vi "质控参数设置.vi"(9 "自动测试量程配置":T1, 10 "质控参数设置":T3) -> (2 "自动测试量程配置输出":T1, 3 "输出簇":T2)   [LabVIEW 2016, in "斯坦道氨氮.lvlib"]
uses:
  <vilib>/Utility/miscctls.llb/LVPointTypeDef.ctl
panel:
  in  "取消":bool
  in  "确定":bool
  in  "总磷标准液标准浓度":dbl
  in  "总磷跨度标准液浓度":dbl
  in  "总磷零点标准液浓度":dbl
  in  "总磷跨度值":dbl
  # "质控量程设置"
  # "监测参数"
  # "氨氮"
  # "跨度值"
  # "mg/L"
  # "零点核查标准液浓度"
  # "mg/L"
  # "跨度核查标准液浓度"
  # "mg/L"
  # "标样核查标准液浓度"
  # "mg/L"
  # "质控参数设置"
  # "监测参数"
  # "氨氮"
  # "跨度值"
  # "零点核查标准液浓度"
  # "跨度核查标准液浓度"
  # "标样核查标准液浓度"
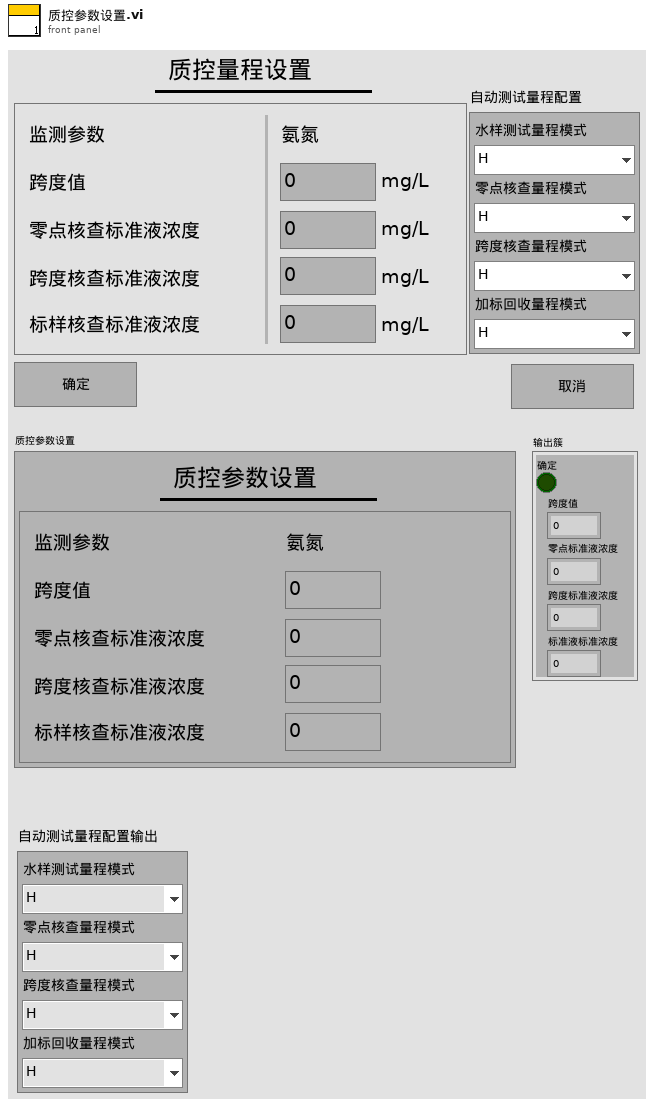
[diagram p1: front panel]
types:
  T1 = cluster{"水样测试量程模式":enum16{"H", "L", "AUTO"}, "空白核查量程模式":enum16{"H", "L", "AUTO"}, "跨度核查量程模式":enum16{"H", "L", "AUTO"}, "加标回收量程模式":enum16{"H", "L", "AUTO"}}
  T2 = cluster{"确定":bool, "跨度值":dbl, "零点标准液浓度":dbl, "跨度标准液浓度":dbl, "标准液标准浓度":dbl}
  T3 = cluster{"总磷跨度值":dbl, "总磷零点标准液浓度":dbl, "总磷跨度标准液浓度":dbl, "总磷标准液标准浓度":dbl}
  T4 = typedef "LVPointTypeDef.ctl" = cluster{"Horizontal":i16, "Vertical":i16}
  T5 = cluster{"确定":bool, "总磷跨度值":dbl, "总磷零点标准液浓度":dbl, "总磷跨度标准液浓度":dbl, "总磷标准液标准浓度":dbl}
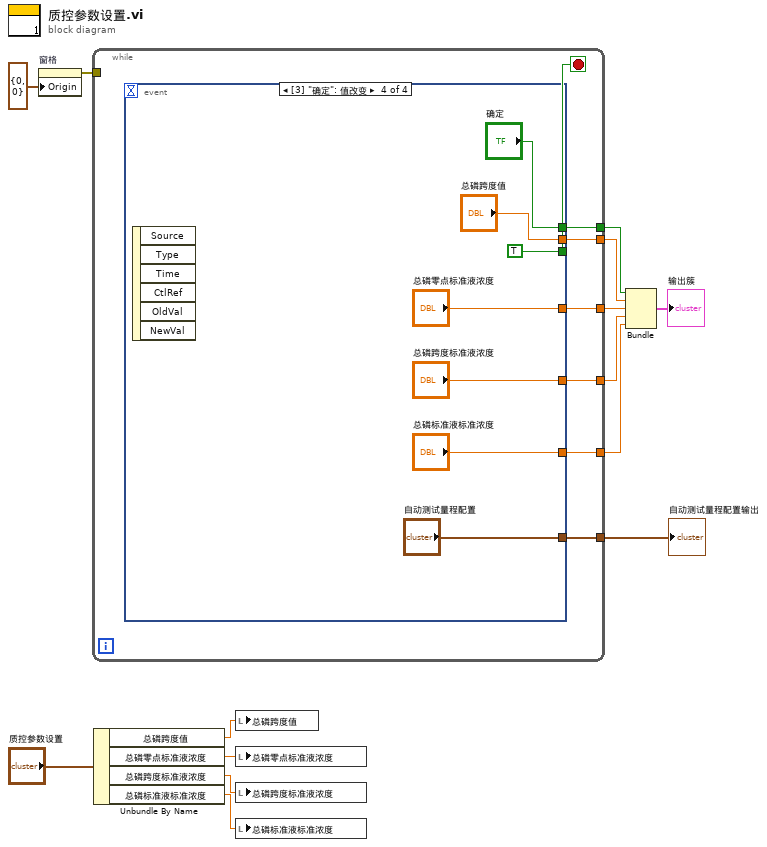
[diagram p0: block diagram]
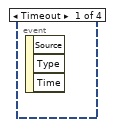
[diagram p2: hidden frame]
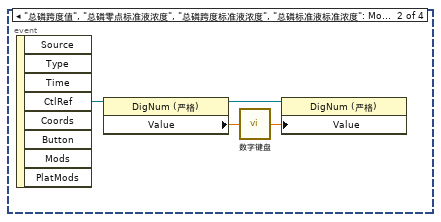
[diagram p3: hidden frame]
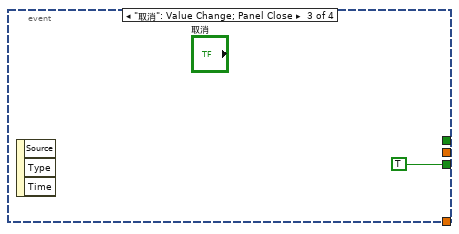
[diagram p4: hidden frame]
diagram:
  n1 = property on="窗格" class="Pane"("Origin"=T4 {"Horizontal"=0, "Vertical"=0} ("原点")) -> (error out=w13:errorcluster)  [unwired: 2 in, 1 out]
  n2 = while {
    tunnel: w13 -> [_]
    tunnel: [w20] -> w12
    tunnel: [w19] -> w11
    tunnel: [w18] -> w10
    tunnel: [w17] -> w9
    tunnel: [w16] -> w8
    tunnel: [w15] -> w1
    stop <- w21 stop-if-true
    n3 = event shown="[3] \"确定\": 值改变" {
      selector: _ -> [_ _ _ _]
      dyn-events: _ -> [_ _ _ _]
      timeout: _ -> [_ _ _ _]
      tunnel: [_ _ TRUE TRUE] -> w21
      tunnel: [_ _ _ "总磷跨度值"] -> w20
      tunnel: [_ _ _ "总磷零点标准液浓度"] -> w19
      tunnel: [_ _ _ "总磷跨度标准液浓度"] -> w18
      tunnel: [_ _ _ "总磷标准液标准浓度"] -> w17
      tunnel: [_ _ _ "确定"] -> w16
      tunnel: [_ _ _ "自动测试量程配置"] -> w15
      event Timeout {
        n4 = event-data() -> ()  [unwired: 1 in, 3 out]
      }
      event "总磷跨度值", "总磷零点标准液浓度", "总磷跨度标准液浓度", "总磷标准液标准浓度": Mouse Down {
        n5 = event-data() -> ("CtlRef"=w25:refnum<vi>)  [unwired: 1 in, 7 out]
        n6 = property class="DigNum (严格)"(reference=w25) -> (reference out=w24:refnum<vi>, "Value"=w23:dbl)  [unwired: 1 in, 1 out]
        n7 = call "数字键盘.vi"("OldNumber"=w23) -> ("NewNumber"=w22:dbl)
        n8 = property class="DigNum (严格)"(reference=w24, "Value"=w22) -> ()  [unwired: 1 in, 2 out]
      }
      event "取消": Value Change; Panel Close {
        n9 = event-data() -> ()  [unwired: 1 in, 3 out]
      }
      event "确定": Value Change {
        n10 = event-data() -> ()  [unwired: 1 in, 6 out]
      }
    }
  }
  "自动测试量程配置输出" <- w1
  n11 = Unbundle By Name("质控参数设置") -> ("总磷跨度值"=w7:dbl, "总磷零点标准液浓度"=w6:dbl, "总磷跨度标准液浓度"=w5:dbl, "总磷标准液标准浓度"=w4:dbl)
  n12 = local write "总磷跨度值"(w7) -> ()
  n13 = local write "总磷零点标准液浓度"(w6) -> ()
  n14 = local write "总磷跨度标准液浓度"(w5) -> ()
  n15 = local write "总磷标准液标准浓度"(w4) -> ()
  n16 = Bundle("确定"=w8, "总磷跨度值"=w12, "总磷零点标准液浓度"=w11, "总磷跨度标准液浓度"=w10, "总磷标准液标准浓度"=w9) -> (→"输出簇":T5)  [unwired: 1 in]
